vi "sharpSensorCalculation.vi"(1 "y":dbl) -> (0 "Numeric 2":dbl)   [LabVIEW 2017]
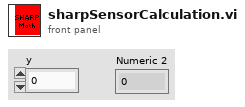
[diagram p1: front panel]
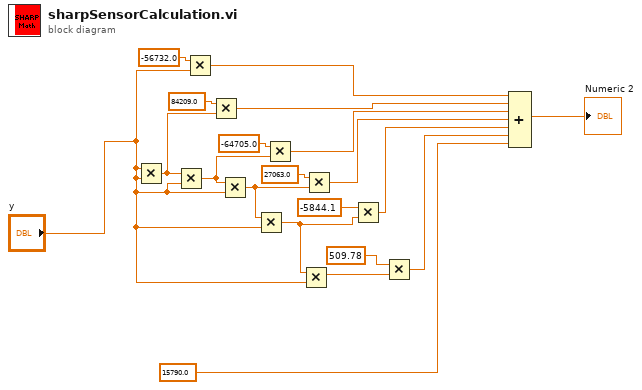
[diagram p0: block diagram]
diagram:
  n1 = Multiply(x="y", y="y") -> (x*y=w20:dbl)
  n2 = Multiply(x=w20, y="y") -> (x*y=w19:dbl)
  n3 = Multiply(x=-56732.0, y="y") -> (x*y=w14:dbl)
  n4 = Multiply(x=84209.0, y=w20) -> (x*y=w13:dbl)
  n5 = Multiply(x=w19, y="y") -> (x*y=w9:dbl)
  n6 = Multiply(x=w9, y="y") -> (x*y=w7:dbl)
  n7 = Multiply(x=-64705.0, y=w19) -> (x*y=w12:dbl)
  n8 = Multiply(x=w7, y="y") -> (x*y=w6:dbl)
  n9 = Multiply(x=27063.0, y=w9) -> (x*y=w11:dbl)
  n10 = Multiply(x=-5844.1, y=w7) -> (x*y=w3:dbl)
  n11 = Multiply(x=509.78, y=w6) -> (x*y=w2:dbl)
  n12 = Compound Arithmetic op=ADD(w14, w13, w12, w11, w3, w2, 15790.0 ("value")) -> (→"Numeric 2":dbl)
